vi "Digital Write Byte.vi"(0 "Arduino Resource":T1, 5 "Start Pin":u8, 9 "Pin Values":bool[](array[boolean]), 11 "error in":errorcluster) -> (4 "Arduino Resource":T1, 15 "error out":errorcluster)   [LabVIEW 2009]
uses:
  <vilib>/LabVIEW Interface for Arduino/LabVIEW Interface for Arduino.lvlib
  <vilib>/LabVIEW Interface for Arduino/Type Defs/Board Type.ctl
  <vilib>/LabVIEW Interface for Arduino/Type Defs/Arduino Resource.ctl
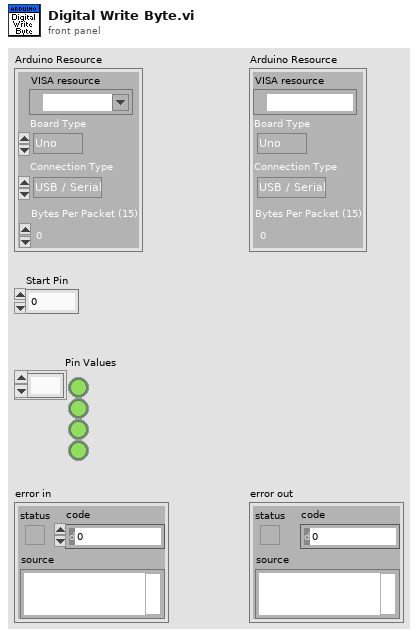
[diagram p1: front panel]
types:
  T1 = typedef "LabVIEW Interface for Arduino.lvlib/Arduino Resource.ctl" = cluster{"VISA resource":refnum<visa-resource-name>, "Board Type":T2, "Connection Type":enum8{"USB / Serial"}, "Bytes Per Packet (15)":u8}
  T2 = typedef "LabVIEW Interface for Arduino.lvlib/Board Type.ctl" = enum16{"Uno", "Dimuelanove w/Atmega 328", "Mega 2560"}
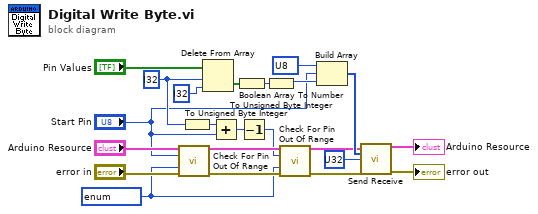
[diagram p0: block diagram]
diagram:
  w7 = enum16{"Analog", "Digital"} ? ("Pin Type")
  w5 = i32 ? ("length")
  n1 = call <vilib>:"Check For Pin Out Of Range.vi"("Arduino Resource"="Arduino Resource", "User Pin Number"="Start Pin", "Pin Type"=w7, "error in"="error in") -> ("Arduino Resource"=w11:T1, "error out"=w10:errorcluster)  [unwired: 10 in]
  n2 = To Unsigned Byte Integer(number=w5) -> (unsigned 8bit integer=w4:u8)
  n3 = Delete From Array(array="Pin Values", length=w5, index=i32 ?) -> (deleted portion=w15:bool[])  [unwired: 1 out]
  n4 = Add(x=w4, y="Start Pin") -> (x+y=w6:u8)
  n5 = Boolean Array To Number(Boolean array=w15) -> (number=w16:u32)
  n6 = Decrement(x=w6) -> (x-1=w3:u8)
  n7 = To Unsigned Byte Integer(number=w16) -> (unsigned 8bit integer=w2:u8)
  n8 = call <vilib>:"Check For Pin Out Of Range.vi"("Arduino Resource"=w11, "User Pin Number"=w3, "Pin Type"=w7, "error in"=w10) -> ("Arduino Resource"=w8:T1, "error out"=w9:errorcluster)  [unwired: 10 in]
  n9 = Build Array(u8 ?, "Start Pin", w2) -> (w22:u8[])
  n10 = call <vilib>:"Send Receive.vi"("Arduino Resource"=w8, "Data"=w22, "Bytes To Read (0)"=u32 ?, "error in"=w9) -> ("Arduino Resource"=→"Arduino Resource":T1, "error out"=→"error out":errorcluster)  [unwired: 9 in, 1 out]
